vi "Timed_muxed_DC_measurement.vi"() -> ()   [LabVIEW 2014]
uses:
  <vilib>/FPGAPlugInAG/PXI-7852R/niLvFpga_Open_PXI-7852R.vi
  <vilib>/rvi/interface/common/dynamic/niFpgaDynamicAddResources.vi
  <vilib>/Utility/error.llb/Error Cluster From Error Code.vi
  <vilib>/rvi/errors/niLvFpgaAdjustHostInterfaceError.vi
  <vilib>/Utility/file.llb/Write To Spreadsheet File (I64).vi
  <vilib>/FPGAPlugInAG/Dynamic/niLvFpga_Close_Dynamic.vi
  <vilib>/measure/maspectr.llb/FFT Power Spectrum and PSD for 1 Chan.vi
  <vilib>/rvi/interface/nirviOpenFPGA/nirviOpenFPGA.xnode
  FPGA Bitfiles/MilitaruDAQ_FPGATarget_MuxedAcquisition_glcrRcw8lng.lvbitx
  Muxed_Acquisition_withDC.vi
  <vilib>/rvi/interface/nirviMethod/nirviMethod.xnode
  <vilib>/rvi/interface/nirviReadWriteControl/nirviReadWriteControl.xnode
  <vilib>/rvi/interface/nirviCloseFPGA/nirviCloseFPGA.xnode
  <vilib>/FPGAPlugInAG/Dynamic/niLvFpga_ReadFifo_Dynamic.vi
  <vilib>/rvi/errors/niLvFpgaMergeErrorWithErrorCode.vi
  NiFpgaLv.dll
  <vilib>/rvi/interface/Simulation/niFpgaSimulationCallBeginRW.vi
  <vilib>/measure/NI_MAPro.lvlib
panel:
  out "Remaining time (s)":u64
  out "Number of Loops":i64
  out "append to file? (new file:F)":bool
  out "x = y?":bool
  in  "Length (s)":dbl
  in  "Number of Elements":u32
  out "Position":waveform(i16)(graph) caption="Dynamic Data Type"
  in  "dB On (F)":bool
  in  "averaging parameters":T1={"averaging mode"=enum."No averaging", "weighting mode"=enum."Exponential", "number of averages"=10} {"number of averages" min=1}
  out "PSD":cluster{"f0":dbl, "df":dbl, "magnitude":dbl[]}(graph) caption="Dynamic Data Type"
  in  "file path (dialog if empty)":path
  in  "append to file? (new file:F)":bool
  in  "Sampling(Ticks)":u32
  out "Sampling Frequency\n(kHz)":dbl
  out "Acquisition Timeout":bool
  out "FIFO timeout":bool
  in  "Acquisition-Channel":i16
  in  "DC sampling":u32
  in  "DC Elements":u32
  out "DC elements remaining":u32
  out "DC-sample [Hz]":dbl
  out "DC":i16[](array[numeric])
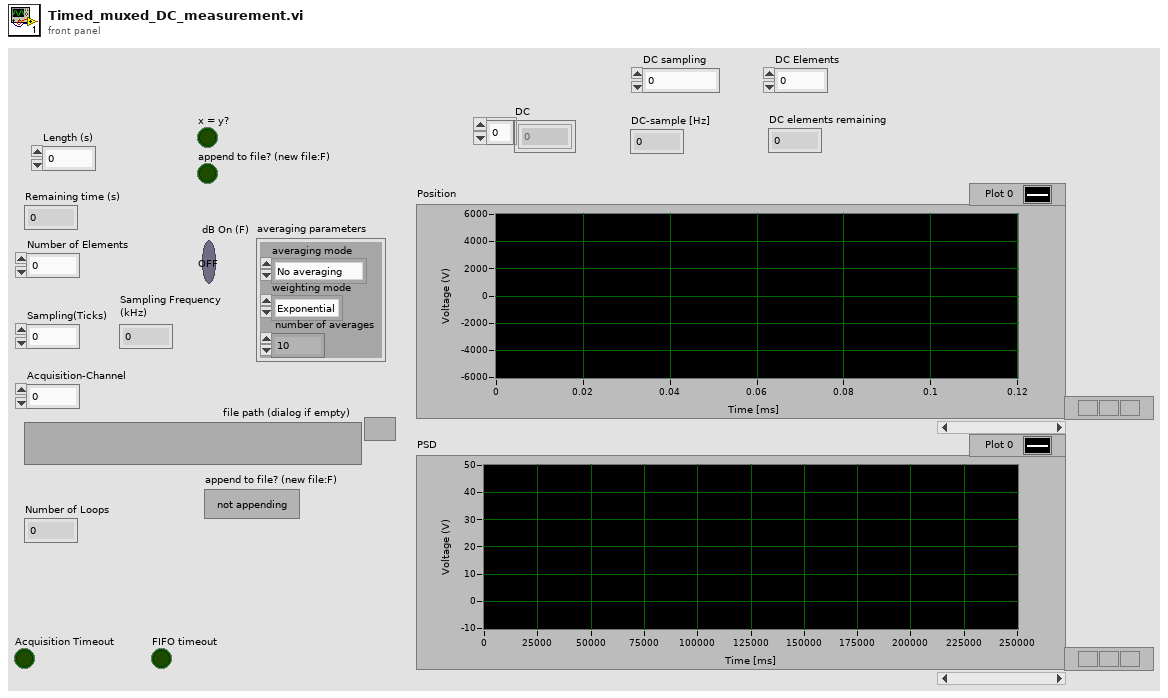
[diagram p1: front panel]
types:
  T1 = cluster{"averaging mode":enum16{"No averaging", "Vector averaging", "RMS averaging", "Peak hold"}, "weighting mode":enum16{"Linear", "Exponential"}, "number of averages":u32}
  T2 = enum16{"open", "replace", "create", "open or create", "replace or create", "replace or create with confirmation"}
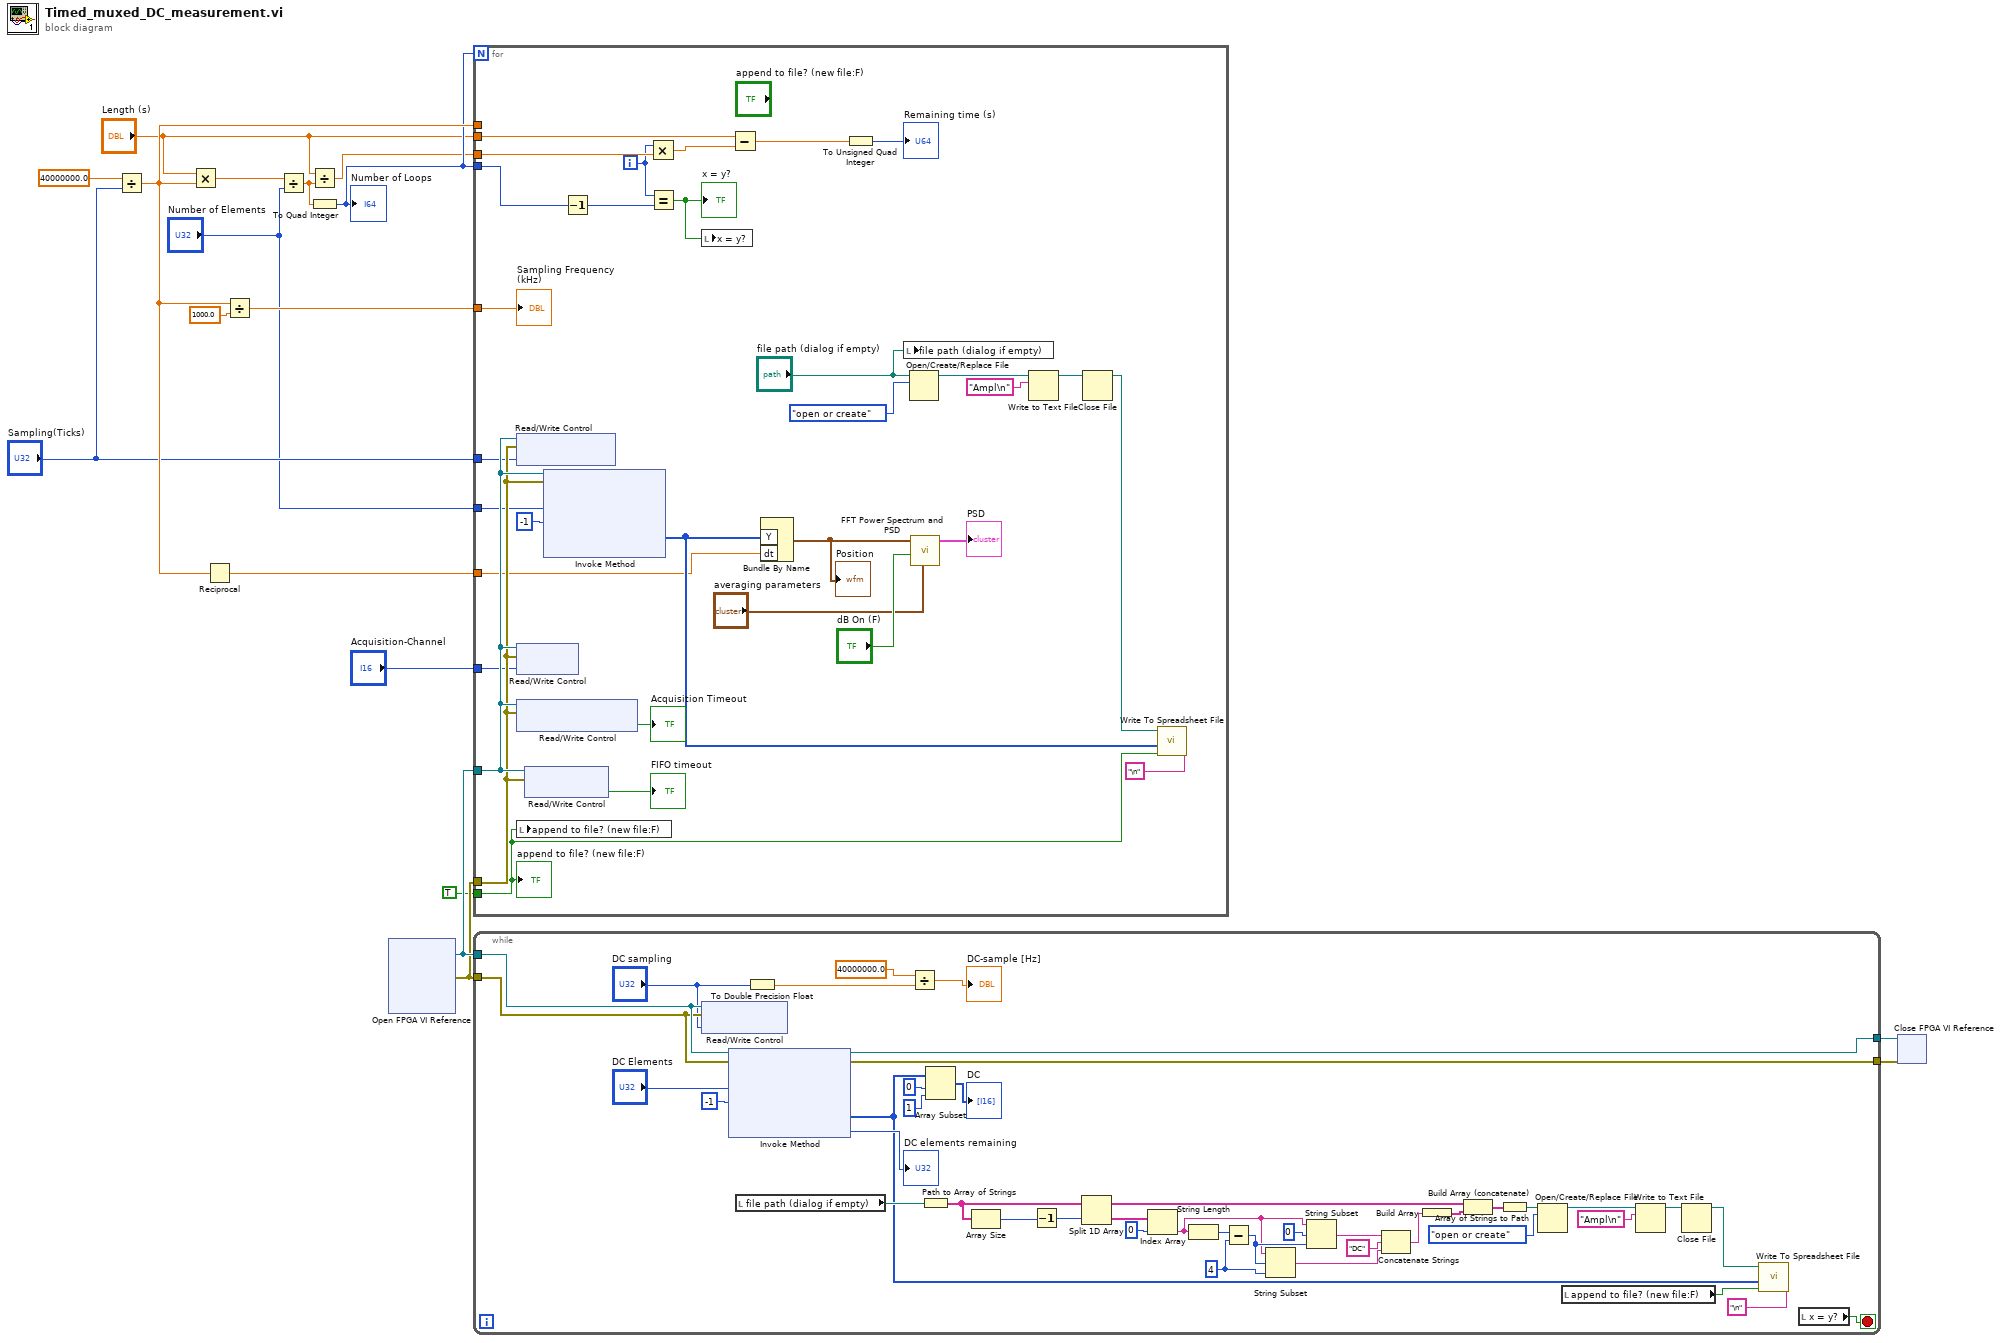
[diagram p0: block diagram]
diagram:
  n1 = Divide(x=40000000.0, y="Sampling(Ticks)") -> (x/y=w11:dbl)
  n2 = Multiply(x="Length (s)", y=w11) -> (x*y=w10:dbl)
  n3 = Reciprocal(x=w11) -> (1/x=w15:dbl)
  n4 = Divide(x=w11, y=1000.0) -> (x/y=w13:dbl)
  n5 = Divide(x=w10, y="Number of Elements") -> (x/y=w3:dbl)
  n6 = Divide(x="Length (s)", y=w3) -> (x/y=w2:dbl)
  n7 = To Quad Integer(1:w3) -> (0:w8:i64)
  "Number of Loops" <- w8
  n8 = xnode "Open FPGA VI Reference"() -> ("FPGA VI Reference Out"=w18:refnum<k20>, "error out"=w17:errorcluster)  [unwired: 2 in]
  n9 = for {
    N: w8 -> [_]
    tunnel: w18 -> [w37]
    tunnel: w17 -> [w36]
    tunnel: "Sampling(Ticks)" -> [w33]
    tunnel: "Number of Elements" -> [w32]
    tunnel: w11 -> [_]
    tunnel: w15 -> [w31]
    tunnel: w13 -> [w30]
    tunnel: "Acquisition-Channel" -> [w29]
    tunnel: TRUE ("append to file? (new file:F)") -> [w28]
    tunnel: w8 -> [w25]
    tunnel: w2 -> [w24]
    tunnel: "Length (s)" -> [w22]
    i -> [w23]
    n10 = xnode "Read/Write Control"("FPGA VI Reference In"=w37, "error in"=w36, "Sampling(Ticks)"=w33) -> ()  [unwired: 2 out]
    n11 = xnode "Read/Write Control"("FPGA VI Reference In"=w37, "error in"=w36, "Numeric"=w29) -> ()  [unwired: 2 out]
    n12 = xnode "Read/Write Control"("FPGA VI Reference In"=w37, "error in"=w36) -> ("Acquisition Timeout"=→"Acquisition Timeout":bool)  [unwired: 2 out]
    n13 = local write "append to file? (new file:F)"(w28) -> ()
    n14 = xnode "Read/Write Control"("FPGA VI Reference In"=w37, "error in"=w36) -> ("FIFO timeout"=→"FIFO timeout":bool)  [unwired: 2 out]
    n15 = xnode "Invoke Method"("FPGA VI Reference In"=w37, "error in"=w36, "Number of Elements"=w32, "Timeout (ms)"=-1) -> ("Data"=w45:i16[])  [unwired: 3 out]
    n16 = Decrement(x=w25) -> (x-1=w26:i64)
    n17 = Multiply(x=w23, y=w24) -> (x*y=w21:dbl)
    n18 = Equal?(x=w23, y=w26) -> (x = y?=w27:bool)
    "x = y?" <- w27
    n19 = local write "x = y?"(w27) -> ()
    n20 = Subtract(x=w22, y=w21) -> (x-y=w20:dbl)
    n21 = Bundle By Name ("Build Waveform")("Y"=w45, "dt"=w31) -> (w49:waveform(i16))  [unwired: 1 in]
    "Position" <- w49
    n22 = To Unsigned Quad Integer(1:w20) -> (0:→"Remaining time (s)":u64)
    n23 = local write "file path (dialog if empty)"("file path (dialog if empty)") -> ()
    n24 = Open/Create/Replace File(file path (use dialog)="file path (dialog if empty)", operation (0:open)=T2."open or create") -> (refnum out=w42:refnum<file>)  [unwired: 4 in, 2 out]
    n25 = call-poly <vilib>:"FFT Power Spectrum and PSD.vi"("averaging parameters"="averaging parameters", "dB On (F)"="dB On (F)", "time signal"=w49) -> ("Power Spectrum / PSD"=→"PSD":cluster{"f0":dbl, "df":dbl, "magnitude":dbl[]})  [unwired: 5 in, 3 out]
    n26 = Write to Text File(file (use dialog)=w42, text="Ampl\n") -> (refnum out=w41:refnum<file>)  [unwired: 2 in, 2 out]
    n27 = Close File(refnum=w41) -> (path=w40:path)  [unwired: 1 in, 1 out]
    n28 = call-poly <vilib>:"Write To Spreadsheet File.vi"("delimiter (\\t)"="\n" ("delimiter (\\t)"), "append to file? (new file:F)"=w28, "1D data"=w45, "file path (dialog if empty)"=w40) -> ()  [unwired: 4 in, 1 out]
    "Sampling Frequency\n(kHz)" <- w30
    "append to file? (new file:F)" <- w28
  }
  n29 = while {
    tunnel: w18 -> [w87]
    tunnel: w17 -> [w86]
    tunnel: [w52] -> w5
    tunnel: [w51] -> w4
    stop <- w53 stop-if-true
    w74 = 4 ("y")
    n30 = xnode "Read/Write Control"("FPGA VI Reference In"=w87, "error in"=w86, "DC-Sampling"="DC sampling") -> ()  [unwired: 2 out]
    n31 = xnode "Invoke Method"("FPGA VI Reference In"=w87, "error in"=w86, "Number of Elements"="DC Elements", "Timeout (ms)"=-1) -> ("FPGA VI Reference Out"=w52:refnum<k20>, "error out"=w51:errorcluster, "Data"=w55:i16[], "Elements Remaining"=→"DC elements remaining":u32)
    n32 = local read "file path (dialog if empty)"() -> (w81:path)
    n33 = To Double Precision Float(number="DC sampling") -> (double precision float=w91:dbl)
    n34 = Divide(x=40000000.0, y=w91) -> (x/y=→"DC-sample [Hz]":dbl)
    n35 = Path to Array of Strings(0:w81) -> (2:w80:string[])  [unwired: 1 out]
    n36 = Array Subset(array=w55, index=0, length=1) -> (→"DC":i16[])
    n37 = Array Size(array=w80) -> (size(s)=w79:i32)
    n38 = Decrement(x=w79) -> (x-1=w78:i32)
    n39 = Split 1D Array(array=w80, index=w78) -> (first subarray=w65:string[], second subarray=w76:string[])
    n40 = Index Array(array=w76, index=0) -> (element=w71:string)
    n41 = String Length(string=w71) -> (length=w75:i32)
    n42 = Subtract(x=w75, y=w74) -> (x-y=w72:i32)
    n43 = String Subset(string=w71, offset (0)=w72, length (rest)=w74) -> (substring=w69:string)
    n44 = String Subset(string=w71, offset (0)=0, length (rest)=w72) -> (substring=w70:string)
    n45 = Concatenate Strings(w70, "DC" ("string"), w69) -> (w67:string)
    n46 = Build Array(w67) -> (w66:string[])
    n47 = Build Array (concatenate)(w65, w66) -> (w64:string[])
    n48 = Array of Strings to Path(0:w64) -> (2:w57:path)  [unwired: 1 in]
    n49 = Open/Create/Replace File(file path (use dialog)=w57, operation (0:open)=T2."open or create") -> (refnum out=w60:refnum<file>)  [unwired: 4 in, 2 out]
    n50 = local read "append to file? (new file:F)"() -> (w56:bool)
    n51 = Write to Text File(file (use dialog)=w60, text="Ampl\n") -> (refnum out=w59:refnum<file>)  [unwired: 2 in, 2 out]
    n52 = Close File(refnum=w59) -> (path=w54:path)  [unwired: 1 in, 1 out]
    n53 = call-poly <vilib>:"Write To Spreadsheet File.vi"("delimiter (\\t)"="\n" ("delimiter (\\t)"), "append to file? (new file:F)"=w56, "1D data"=w55, "file path (dialog if empty)"=w54) -> ()  [unwired: 4 in, 1 out]
    n54 = local read "x = y?"() -> (w53:bool)
  }
  n55 = xnode "Close FPGA VI Reference"("FPGA VI Reference In"=w5, "error in"=w4) -> ()  [unwired: 1 out]
